vi "Drive_utils_LimitAngle.vi"(3 "Minimum Angle":dbl, 4 "Max Angle Per Iteration":dbl=0.1745, 5 "Angle":dbl, 6 "distance in":dbl) -> (1 "Angle out":dbl, 2 "distance out":dbl)   [LabVIEW 2009, in "Drive.lvlib" / "Drive_Utils.lvlib"]
uses:
  Drive_Utils.lvlib
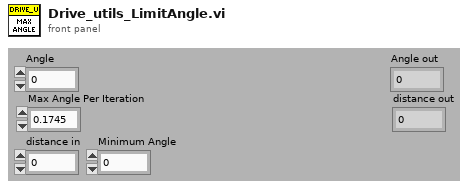
[diagram p1: front panel]
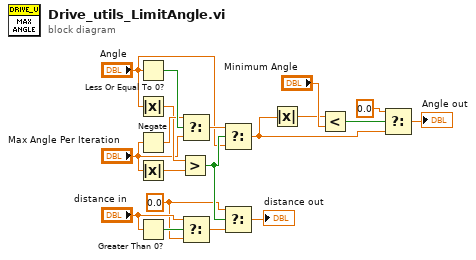
[diagram p0: block diagram]
diagram:
  w1 = 0.0 ("t")
  n1 = Less Or Equal To 0?(x="Angle") -> (x <= 0?=w17:bool)
  n2 = Absolute Value(x="Angle") -> (abs(x)=w13:dbl)
  n3 = Negate(x="Max Angle Per Iteration") -> (-x=w16:dbl)
  n4 = Absolute Value(x="Max Angle Per Iteration") -> (abs(x)=w11:dbl)
  n5 = Greater Than 0?(x="distance in") -> (x > 0?=w2:bool)
  n6 = Greater?(x=w13, y=w11) -> (0:w19:bool)
  n7 = Select(t=w16, s=w17, f="Max Angle Per Iteration") -> (s? t:f=w15:dbl)
  n8 = Select(t="distance in", s=w2, f=w1) -> (s? t:f=w4:dbl)
  n9 = Select(t=w15, s=w19, f="Angle") -> (s? t:f=w6:dbl)
  n10 = Select(t=w1, s=w19, f=w4) -> (s? t:f=→"distance out":dbl)
  n11 = Absolute Value(x=w6) -> (abs(x)=w5:dbl)
  n12 = Less?(x=w5, y="Minimum Angle") -> (x < y?=w10:bool)
  n13 = Select(t=0.0, s=w10, f=w6) -> (s? t:f=→"Angle out":dbl)
